vi "Queue monitor FVG.vi"(6 "max elements (150)":i32=150, 7 "Akcja (SET)":T1, 8 "error in (no error)":errorcluster, 11 "queue in":refnum<queue>) -> (0 "error out":errorcluster, 4 "# elements in szybka":i32)   [LabVIEW 2014]
doc: "Use this template to build a VI to use as a subVI."
uses:
  Kontrolki/Przetwarzanie/Kanaly.ctl
  Kontrolki/FVGs/FVG akcje podstawowa.ctl
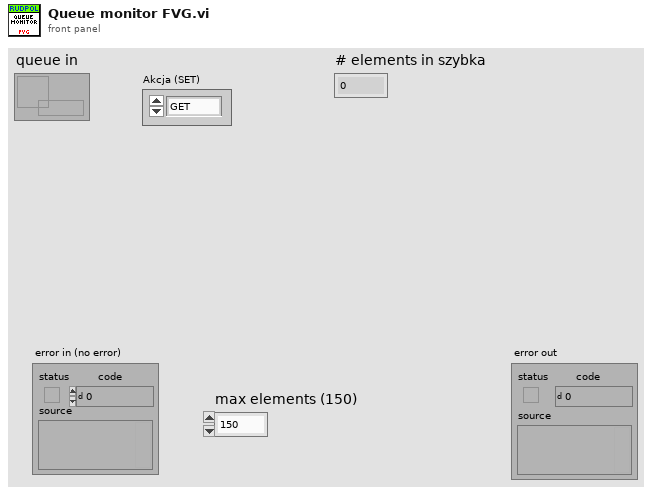
[diagram p1: front panel]
types:
  T1 = typedef "FVG akcje podstawowa.ctl" = enum16{"GET", "SET"}
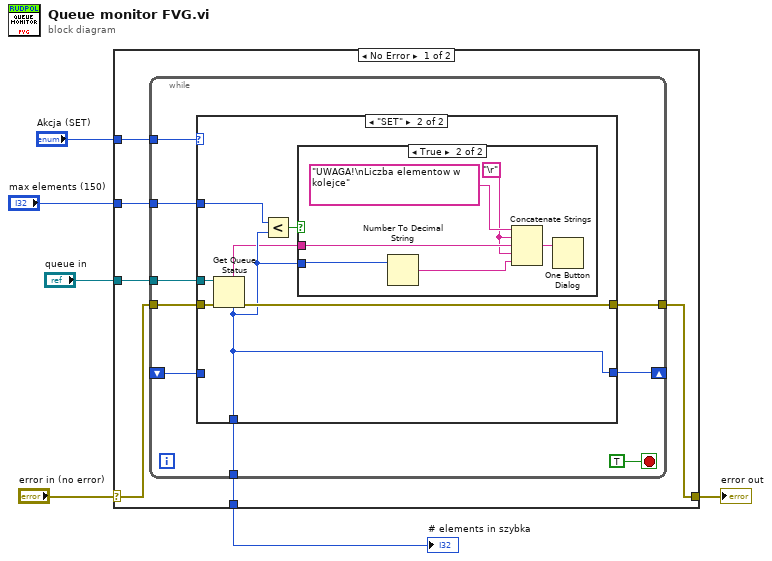
[diagram p0: block diagram]
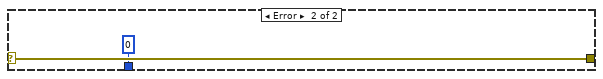
[diagram p4: hidden frame]
diagram:
  n1 = case shown="No Error" "error in (no error)" {
    selector: "error in (no error)" -> [w12 w38]
    tunnel: [w9 w38] -> w5
    tunnel: "Akcja (SET)" -> [w11 _]
    tunnel: "queue in" -> [w10 _]
    tunnel: "max elements (150)" -> [w8 _]
    tunnel: [w7 0 ("# elements in queue")] -> w1
    frame No Error {
      n2 = while {
        tunnel: w12 -> [w21]
        tunnel: w11 -> [w20]
        tunnel: w10 -> [w19]
        tunnel: [w18] -> w9
        tunnel: w8 -> [w16]
        tunnel: [w15] -> w7
        shift-right: [w14] -> _
        shift-left: _ -> [w13]
        stop <- TRUE stop-if-true
        n3 = case shown="\"SET\"" w20 {
          tunnel: w21 -> [w23 w30]
          tunnel: w19 -> [_ w29]
          tunnel: [w23 w28] -> w18
          tunnel: w16 -> [_ w27]
          tunnel: [w22 w25] -> w15
          tunnel: [w22 w25] -> w14
          tunnel: w13 -> [w22 _]
          frame "GET", Default {
          }
          frame "SET" {
            n4 = Get Queue Status(queue=w29, error in (no error)=w30) -> (queue name=w24:string, error out=w28:errorcluster, # elements in queue=w25:i32)  [unwired: 1 in, 5 out]
            n5 = Less?(x=w27, y=w25) -> (x < y?=w26:bool)
            n6 = case shown="True" w26 {
              tunnel: w25 -> [_ w34]
              tunnel: w24 -> [_ w33]
              frame False {
              }
              frame True {
                w32 = "\r"
                n7 = Number To Decimal String(number=w34) -> (decimal integer string=w31:string)  [unwired: 1 in]
                n8 = Concatenate Strings("UWAGA!\nLiczba elementow w kolejce" ("message"), w32, w33, w32, w31) -> (w35:string)
                n9 = One Button Dialog(message=w35) -> ()  [unwired: 1 in, 1 out]
              }
            }
          }
        }
      }
    }
    frame Error {
    }
  }
  "error out" <- w5
  "# elements in szybka" <- w1
